vi "Find Local Msg Set.vi"(11 "Core Actor in":refnum<class "Core Actor.lvclass">) -> (3 "Core Actor out":refnum<class "Core Actor.lvclass">)   [LabVIEW 2025, in "jettl.lvlib" / "Actor.lvlib" / "Core Actor.lvclass"]
uses:
  Core Actor.lvclass
  Core Actor.lvclass/Core Actor.ctl
  C:/git/jettl/src/jettl/jettl/Actor/Core Actor/Core Actor.lvclass
  C:/git/jettl/src/jettl/jettl/Actor/Actor/Actor.lvclass
  C:/git/jettl/src/jettl/jettl/Stop Msg/Stop/Stop.lvclass
  C:/git/jettl/src/jettl/jettl/Stopped Msg/Stopped/Stopped.lvclass
  jettl.lvlib
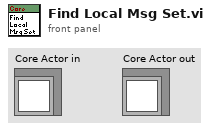
[diagram p1: front panel]
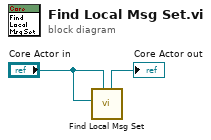
[diagram p0: block diagram]
diagram:
  n1 = call "Find Local Msg Set.vi"("Actor in"="Core Actor in", "X Actor.lvclass"="Core Actor in") -> ("Actor out"=→"Core Actor out":refnum<class "Core Actor.lvclass">)  [unwired: 9 in]
